vi "DAC Save Results.vi"(8 "error in":errorcluster, 9 "Log Details?":bool, 10 "tdms file":refnum<k34>, 11 "DAC CS Humid in":refnum<class "DAC CS Humid.lvclass">) -> (0 "error out":errorcluster)   [LabVIEW 2019, in "DAC.lvlib" / "DAC CS Humid.lvclass"]
uses:
  DAC CS Humid.lvclass
  C:/Users/krio/Documents/LV_Projects/test-stand/App/DAC/DAC.lvclass
  DAC.lvclass/DAC.ctl
  DAC CS Humid.lvclass/DAC CS Humid.ctl
  DAC.lvclass
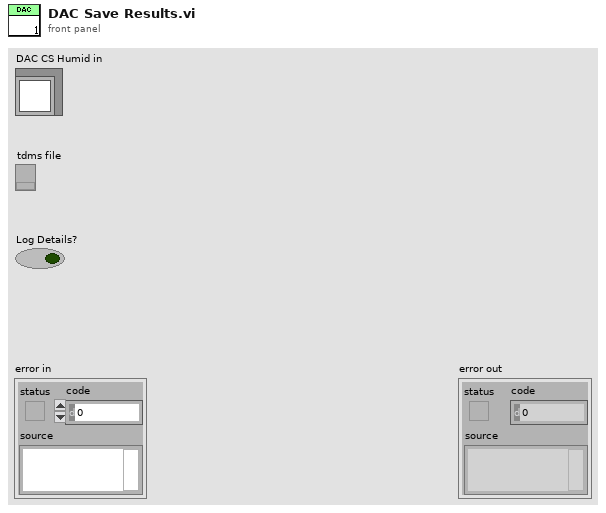
[diagram p1: front panel]
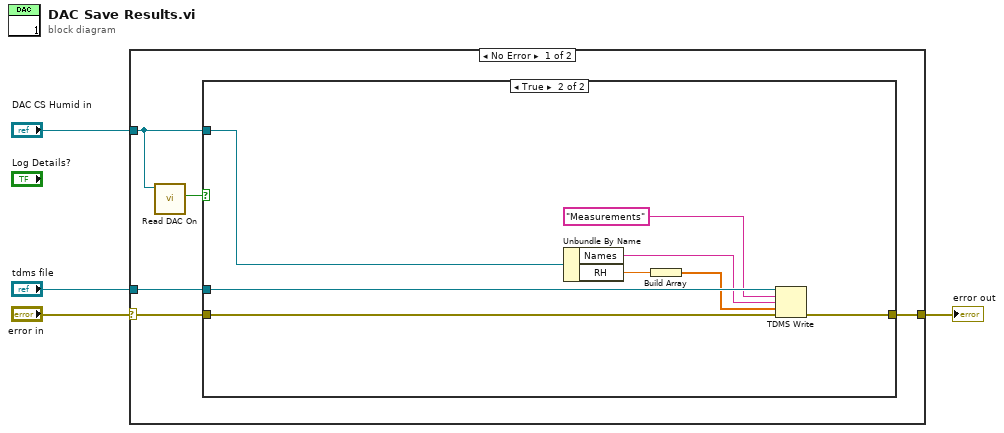
[diagram p0: block diagram]
diagram:
  n1 = case shown="No Error" "error in" {
    selector: "error in" -> [w6 w19]
    tunnel: "DAC CS Humid in" -> [w9 _]
    tunnel: "tdms file" -> [w7 _]
    tunnel: [w5 w19] -> w1
    frame No Error {
      n2 = call "Read DAC On.vi"("DAC in"=w9) -> ("DAC On"=w8:bool)  [unwired: 8 in, 2 out]
      n3 = case shown="True" w8 {
        tunnel: w9 -> [_ w18]
        tunnel: w7 -> [_ w17]
        tunnel: w6 -> [w10 w14]
        tunnel: [w10 w16] -> w5
        frame False {
        }
        frame True {
          n4 = Unbundle By Name(w18) -> ("Names"=w12:string, "RH"=w13:dbl)
          n5 = Build Array(w13) -> (w11:dbl[])
          n6 = TDMS Write(0:w17, 5:"Measurements" ("group name in (Untitled)"), 7:w12, 9:w11, 11:w14) -> (15:w16:errorcluster)  [unwired: 1 in, 3 out]
        }
      }
    }
    frame Error {
    }
  }
  "error out" <- w1
